vi "SerialCommError.vi"(0 "VISA IN":refnum<visa-resource-name>, 11 "error IN":errorcluster) -> (4 "VISA OUT":refnum<visa-resource-name>, 8 "Error":bool, 15 "error OUT":errorcluster)   [LabVIEW 2011]
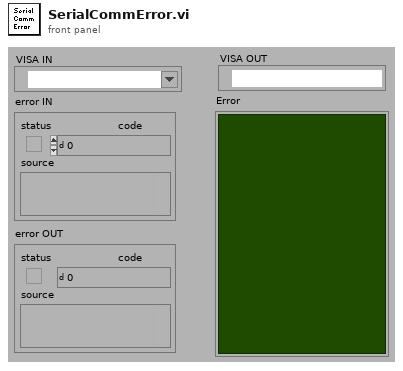
[diagram p1: front panel]
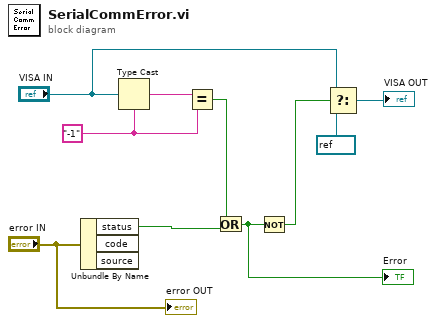
[diagram p0: block diagram]
diagram:
  w8 = "-1"
  n1 = Unbundle By Name("error IN") -> ("status"=w6:bool)  [unwired: 2 out]
  n2 = Type Cast(type=w8, x="VISA IN") -> (*(type *) &x=w9:string)
  n3 = Equal?(x=w9, y=w8) -> (x = y?=w7:bool)
  n4 = Or(x=w7, y=w6) -> (x .or. y?=w1:bool)
  "Error" <- w1
  n5 = Not(x=w1) -> (.not. x?=w5:bool)
  n6 = Select(t="VISA IN", s=w5, f=refnum<visa-resource-name> "-1") -> (s? t:f=→"VISA OUT":refnum<visa-resource-name>)
  "error OUT" <- "error IN"
